vi "Stop Log.vi"(8 "error in (no error)":errorcluster, 11 "LoggingManager in":refnum<class "LoggingManager.lvclass">) -> (0 "error out":errorcluster, 3 "LoggingManager out":refnum<class "LoggingManager.lvclass">)   [LabVIEW 2020, in "VolatusDataLogger.lvlib" / "LoggingManager.lvclass"]
uses:
  LoggingManager.lvclass
  LoggingManager.lvclass/LoggingManager.ctl
  LoggingHandler Messages/Stop Log Msg/Stop Log Msg.lvclass
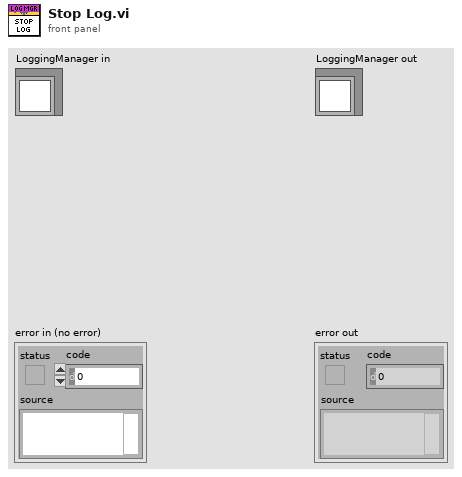
[diagram p1: front panel]
types:
  T1 = map{string, refnum<class "Message Enqueuer.lvclass">}
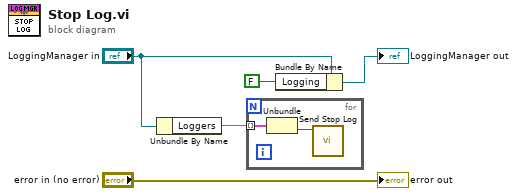
[diagram p0: block diagram]
diagram:
  n1 = Unbundle By Name("LoggingManager in") -> ("Loggers"=w4:T1)
  n2 = for {
    tunnel: w4 -> [w7] mode=indexing
    n3 = Unbundle(w7) -> ("EnQr"=w6:refnum<class "Message Enqueuer.lvclass">)  [unwired: 1 out]
    n4 = call "Send Stop Log.vi"("Message Enqueuer"=w6) -> ()  [unwired: 9 in, 2 out]
  }
  n5 = Bundle By Name(cluster="LoggingManager in", "Logging"=FALSE) -> (→"LoggingManager out":refnum<class "LoggingManager.lvclass">)
  "error out" <- "error in (no error)"
